vi "基于LabVIEW的多点温度监测系统上位机软件.vi"() -> ()   [LabVIEW 2022 SP3]
uses:
  <vilib>/Instr/_visa.llb/VISA Configure Serial Port (Instr).vi
panel:
  out "获取从机01返回的原始数据包":string
  in  "选择从机":u16(ring)=1 items=["从机01"=1, "从机02"=2]
  out "地址02":dbl[][](graph)
  out "地址01":dbl[][](graph)
  out "提取的第四路温度原始数据":string
  out "提取的第三路温度原始数据":string
  out "提取的第二路温度原始数据":string
  out "提取的第一路温度原始数据":string
  out "提取的第四路温度原始数据":string
  out "提取的第三路温度原始数据":string
  out "提取的第二路温度原始数据":string
  out "提取的第一路温度原始数据":string
  out "第一路温度值":dbl[](array[numeric])
  in  "停止采集":bool
  out "所有测量记录":string[][](table)
  out "第一路温度值":dbl[](array[numeric])
  out "获取从机02返回的原始数据包":string
  in  "发送命令":string
  in  "波特率":u32=9600 caption="波特率(9600)"
  in  "选择串口":refnum<visa-resource-name>
  # "从机地址01："
  # "第二路温度值"
  # "第三路温度值"
  # "第四路温度值"
  # "从机地址02："
  # "第二路温度值"
  # "第三路温度值"
  # "第四路温度值"
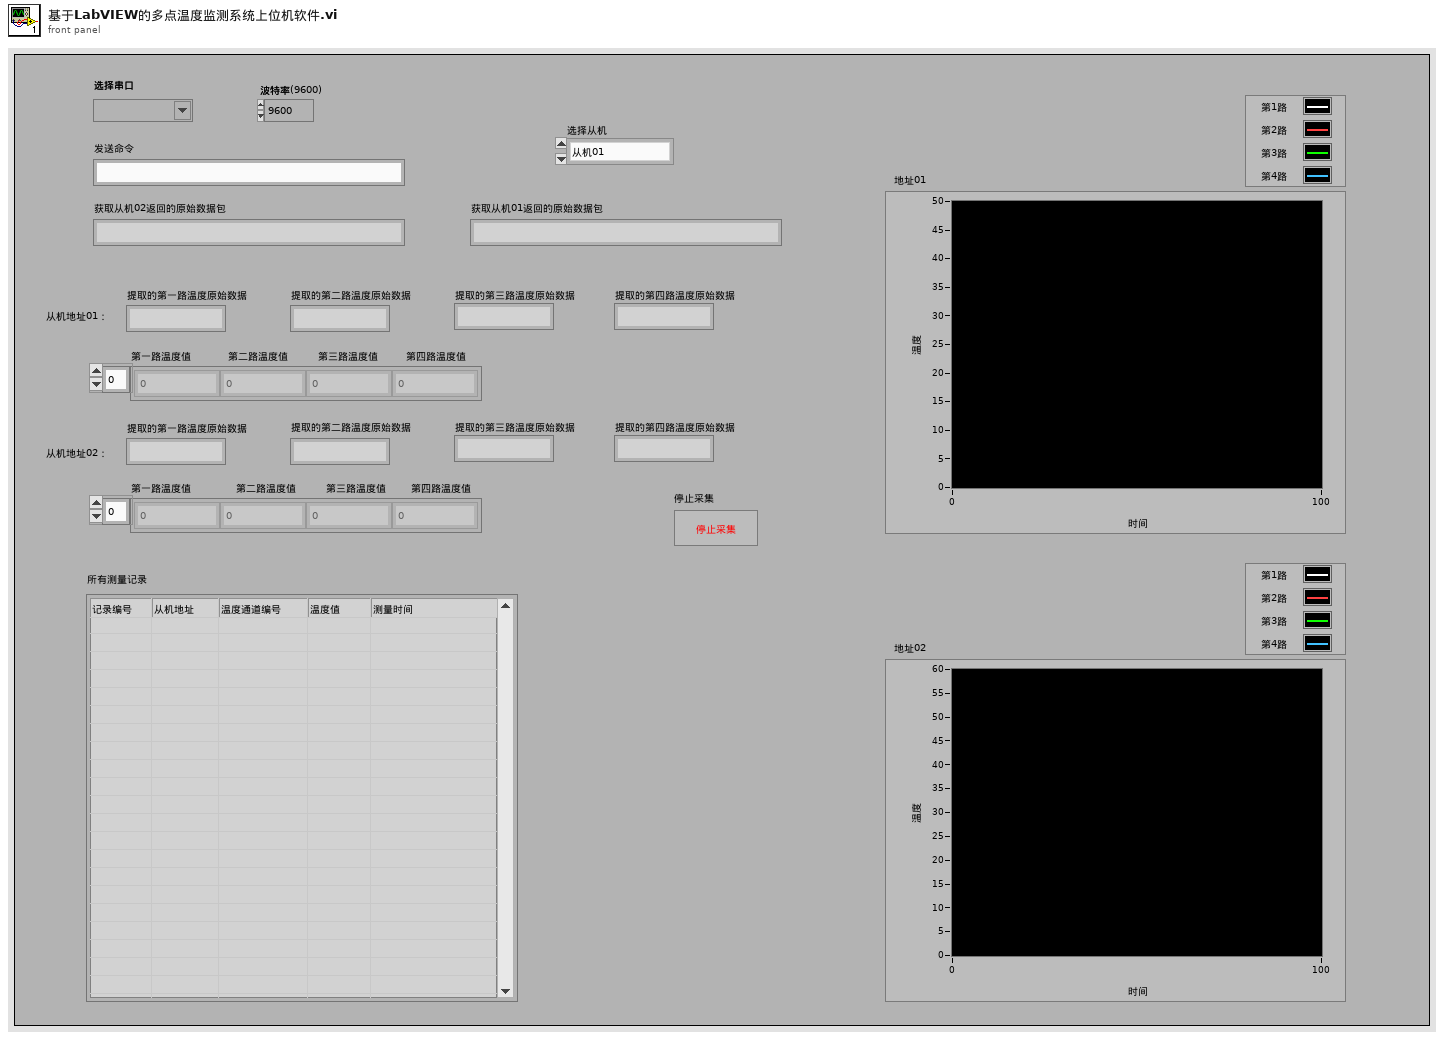
[diagram p1: front panel]
types:
  T1 = typedef "NI_Matrix.lvlib/RealMatrix.ctl" = dbl[][]
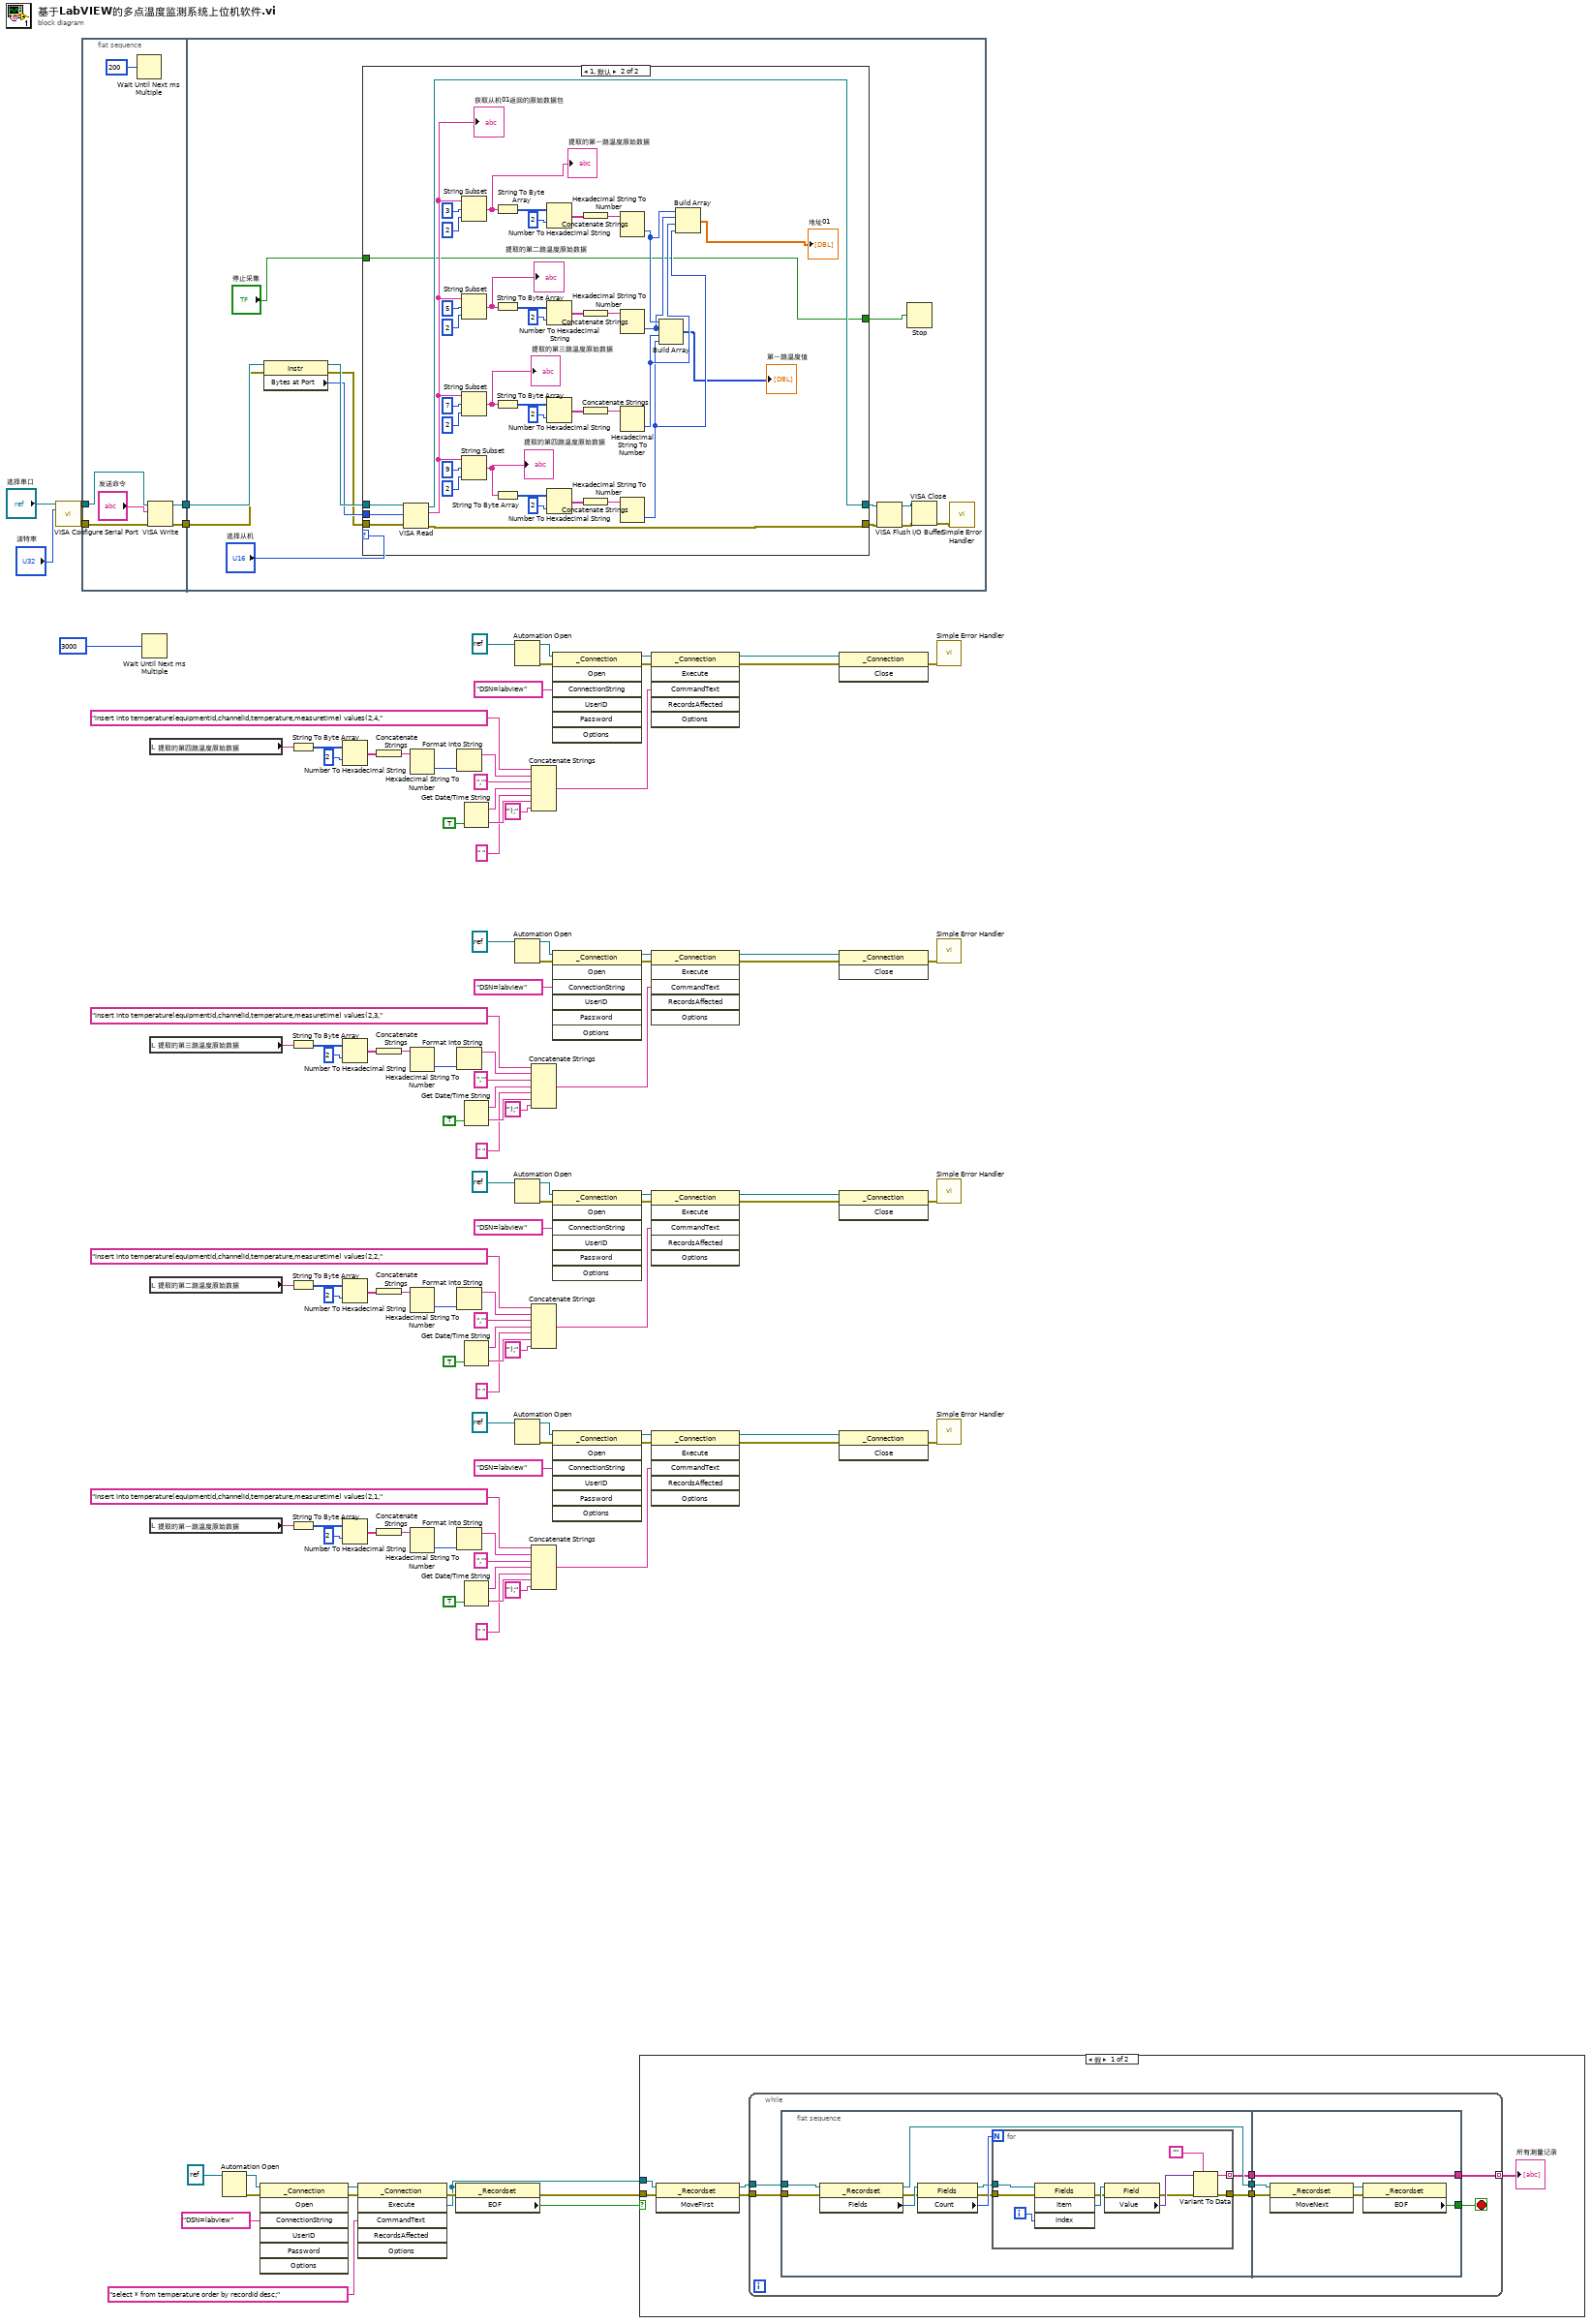
[diagram p0: block diagram]
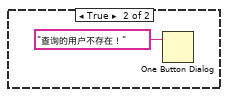
[diagram p2: hidden frame]
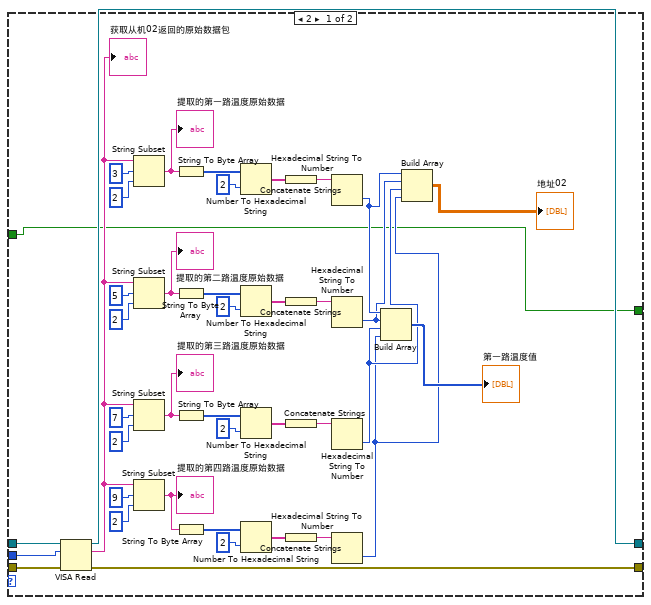
[diagram p3: hidden frame]
diagram:
  n1 = call-poly "VISA Configure Serial Port"("VISA resource name"="选择串口", "baud rate (9600)"="波特率") -> ("VISA resource name out"=w112:refnum<visa-resource-name>, "error out"=w111:errorcluster)  [unwired: 12 in]
  n2 = flat-sequence {
    tunnel: w112 -> [w119]
    tunnel: w111 -> [w118]
    tunnel: [w116] -> w110
    tunnel: [w115] -> w109
    tunnel: w110 -> [w133]
    tunnel: w109 -> [w132]
    frame #0 {
      n3 = Wait Until Next ms Multiple(millisecond multiple=u32 200 ("毫秒倍数")) -> ()  [unwired: 1 out]
      n4 = VISA Write(VISA resource name=w119, write buffer="发送命令", error in (no error)=w118) -> (VISA resource name out=w116:refnum<visa-resource-name>, error out=w115:errorcluster)  [unwired: 1 out]
    }
    frame #1 {
      n5 = property class="Instr"(reference=w133, error in=w132) -> (reference out=w131:refnum<visa-resource-name>, error out=w129:errorcluster, "Bytes at Port"=w130:u32)
      n6 = case shown="1, 默认" "选择从机" {
        tunnel: w131 -> [w174 w178]
        tunnel: w130 -> [w173 w177]
        tunnel: w129 -> [w172 w187]
        tunnel: [w164 w185] -> w125
        tunnel: [w163 w186] -> w124
        tunnel: [w134 w175] -> w121
        tunnel: "停止采集" -> [w134 w175]
        frame 2 {
          n7 = VISA Read(VISA resource name=w174, byte count=w173, error in (no error)=w172) -> (VISA resource name out=w164:refnum<visa-resource-name>, read buffer=w142:string, error out=w163:errorcluster)  [unwired: 1 out]
          "获取从机02返回的原始数据包" <- w142
          n8 = String Subset(string=w142, offset (0)=3 ("偏移量(0)"), length (rest)=2 ("长度（剩余）")) -> (substring=w169:string)
          "提取的第一路温度原始数据" <- w169
          n9 = String Subset(string=w142, offset (0)=5 ("偏移量(0)"), length (rest)=2 ("长度（剩余）")) -> (substring=w160:string)
          "提取的第二路温度原始数据" <- w160
          n10 = String Subset(string=w142, offset (0)=7 ("偏移量(0)"), length (rest)=2 ("长度（剩余）")) -> (substring=w153:string)
          "提取的第三路温度原始数据" <- w153
          n11 = String Subset(string=w142, offset (0)=9 ("偏移量(0)"), length (rest)=2 ("长度（剩余）")) -> (substring=w147:string)
          "提取的第四路温度原始数据" <- w147
          n12 = String To Byte Array(string=w169) -> (unsigned byte array=w168:u8[])
          n13 = String To Byte Array(string=w160) -> (unsigned byte array=w159:u8[])
          n14 = String To Byte Array(string=w153) -> (unsigned byte array=w152:u8[])
          n15 = String To Byte Array(string=w147) -> (unsigned byte array=w146:u8[])
          n16 = Number To Hexadecimal String(1:i16 2 ("宽度(-)"), 2:w168) -> (0:w166:string[])
          n17 = Number To Hexadecimal String(1:i16 2 ("宽度(-)"), 2:w159) -> (0:w157:string[])
          n18 = Number To Hexadecimal String(1:i16 2 ("宽度(-)"), 2:w152) -> (0:w150:string[])
          n19 = Number To Hexadecimal String(1:i16 2 ("宽度(-)"), 2:w146) -> (0:w144:string[])
          n20 = Concatenate Strings(w166) -> (w165:string)
          n21 = Concatenate Strings(w157) -> (w156:string)
          n22 = Concatenate Strings(w150) -> (w149:string)
          n23 = Concatenate Strings(w144) -> (w143:string)
          n24 = Hexadecimal String To Number(string=w165) -> (number=w138:u32)  [unwired: 2 in, 1 out]
          n25 = Hexadecimal String To Number(string=w156) -> (number=w137:u32)  [unwired: 2 in, 1 out]
          n26 = Hexadecimal String To Number(string=w149) -> (number=w136:u32)  [unwired: 2 in, 1 out]
          n27 = Hexadecimal String To Number(string=w143) -> (number=w135:u32)  [unwired: 2 in, 1 out]
          n28 = Build Array(w138, w137, w136, w135) -> (→"第一路温度值":u32[])
          n29 = Build Array(w138, w137, w136, w135) -> (→"地址02":T1)
        }
        frame 1, Default {
          n30 = VISA Read(VISA resource name=w178, byte count=w177, error in (no error)=w187) -> (VISA resource name out=w185:refnum<visa-resource-name>, read buffer=w176:string, error out=w186:errorcluster)  [unwired: 1 out]
          "获取从机01返回的原始数据包" <- w176
          n31 = String Subset(string=w176, offset (0)=3 ("偏移量(0)"), length (rest)=2 ("长度（剩余）")) -> (substring=w181:string)
          "提取的第一路温度原始数据" <- w181
          n32 = String Subset(string=w176, offset (0)=5 ("偏移量(0)"), length (rest)=2 ("长度（剩余）")) -> (substring=w182:string)
          "提取的第二路温度原始数据" <- w182
          n33 = String Subset(string=w176, offset (0)=7 ("偏移量(0)"), length (rest)=2 ("长度（剩余）")) -> (substring=w183:string)
          "提取的第三路温度原始数据" <- w183
          n34 = String Subset(string=w176, offset (0)=9 ("偏移量(0)"), length (rest)=2 ("长度（剩余）")) -> (substring=w184:string)
          "提取的第四路温度原始数据" <- w184
          n35 = String To Byte Array(string=w181) -> (unsigned byte array=w213:u8[])
          n36 = String To Byte Array(string=w182) -> (unsigned byte array=w207:u8[])
          n37 = String To Byte Array(string=w183) -> (unsigned byte array=w201:u8[])
          n38 = String To Byte Array(string=w184) -> (unsigned byte array=w196:u8[])
          n39 = Number To Hexadecimal String(1:i16 2 ("宽度(-)"), 2:w213) -> (0:w211:string[])
          n40 = Number To Hexadecimal String(1:i16 2 ("宽度(-)"), 2:w207) -> (0:w205:string[])
          n41 = Number To Hexadecimal String(1:i16 2 ("宽度(-)"), 2:w201) -> (0:w199:string[])
          n42 = Number To Hexadecimal String(1:i16 2 ("宽度(-)"), 2:w196) -> (0:w194:string[])
          n43 = Concatenate Strings(w211) -> (w210:string)
          n44 = Concatenate Strings(w205) -> (w204:string)
          n45 = Concatenate Strings(w199) -> (w198:string)
          n46 = Concatenate Strings(w194) -> (w193:string)
          n47 = Hexadecimal String To Number(string=w210) -> (number=w191:u32)  [unwired: 2 in, 1 out]
          n48 = Hexadecimal String To Number(string=w204) -> (number=w190:u32)  [unwired: 2 in, 1 out]
          n49 = Hexadecimal String To Number(string=w198) -> (number=w189:u32)  [unwired: 2 in, 1 out]
          n50 = Hexadecimal String To Number(string=w193) -> (number=w188:u32)  [unwired: 2 in, 1 out]
          n51 = Build Array(w191, w190, w189, w188) -> (→"第一路温度值":u32[])
          n52 = Build Array(w191, w190, w189, w188) -> (→"地址01":T1)
        }
      }
      n53 = VISA Flush I/O Buffer(VISA resource name=w125, error in (no error)=w124) -> (VISA resource name out=w126:refnum<visa-resource-name>, error out=w127:errorcluster)  [unwired: 1 in]
      n54 = Stop(stop? (T)=w121) -> ()
      n55 = VISA Close(VISA resource name=w126, error in (no error)=w127) -> (error out=w128:errorcluster)
      n56 = call <vilib>:"Simple Error Handler.vi"("error in (no error)"=w128) -> ()  [unwired: 4 in, 5 out]
    }
  }
  n57 = Wait Until Next ms Multiple(millisecond multiple=3000) -> ()  [unwired: 1 out]
  n58 = local read "提取的第四路温度原始数据"() -> (w2:string)
  n59 = local read "提取的第三路温度原始数据"() -> (w3:string)
  n60 = local read "提取的第二路温度原始数据"() -> (w44:string)
  n61 = local read "提取的第一路温度原始数据"() -> (w65:string)
  n62 = Automation Open(Automation Refnum=refnum<k7> refnum ("ADODB._Connection")) -> (Automation Refnum=w107:refnum<k7>, error out=w106:errorcluster)  [unwired: 3 in]
  n63 = invoke class="_Connection" method="Open"(reference=w107, error in=w106, "ConnectionString"="DSN=labview") -> (reference out=w104:refnum<k7>, error out=w103:errorcluster)  [unwired: 4 in, 5 out]
  n64 = String To Byte Array(string=w2) -> (unsigned byte array=w20:u8[])
  n65 = String To Byte Array(string=w3) -> (unsigned byte array=w40:u8[])
  n66 = String To Byte Array(string=w44) -> (unsigned byte array=w61:u8[])
  n67 = String To Byte Array(string=w65) -> (unsigned byte array=w82:u8[])
  n68 = Number To Hexadecimal String(1:i16 2 ("宽度(-)"), 2:w20) -> (0:w21:string[])
  n69 = Number To Hexadecimal String(1:i16 2 ("宽度(-)"), 2:w40) -> (0:w41:string[])
  n70 = Number To Hexadecimal String(1:i16 2 ("宽度(-)"), 2:w61) -> (0:w62:string[])
  n71 = Number To Hexadecimal String(1:i16 2 ("宽度(-)"), 2:w82) -> (0:w83:string[])
  n72 = invoke class="_Connection" method="Execute"(reference=w104, error in=w103, "CommandText"="select * from temperature order by recordid desc;") -> (error out=w101:errorcluster, "Execute"=w99:refnum<k7>)  [unwired: 3 in, 4 out]
  n73 = Concatenate Strings(w21) -> (w22:string)
  n74 = Concatenate Strings(w41) -> (w42:string)
  n75 = Concatenate Strings(w62) -> (w63:string)
  n76 = Concatenate Strings(w83) -> (w84:string)
  n77 = Hexadecimal String To Number(string=w22) -> (number=w23:u32)  [unwired: 2 in, 1 out]
  n78 = Hexadecimal String To Number(string=w42) -> (number=w43:u32)  [unwired: 2 in, 1 out]
  n79 = Hexadecimal String To Number(string=w63) -> (number=w64:u32)  [unwired: 2 in, 1 out]
  n80 = Hexadecimal String To Number(string=w84) -> (number=w85:u32)  [unwired: 2 in, 1 out]
  n81 = property class="_Recordset"(reference=w99, error in=w101) -> (error out=w98:errorcluster, "EOF"=w100:bool)  [unwired: 1 out]
  n82 = Format Into String(w23) -> (resulting string=w19:string)  [unwired: 3 in, 1 out]
  n83 = Format Into String(w43) -> (resulting string=w39:string)  [unwired: 3 in, 1 out]
  n84 = Format Into String(w64) -> (resulting string=w60:string)  [unwired: 3 in, 1 out]
  n85 = Format Into String(w85) -> (resulting string=w81:string)  [unwired: 3 in, 1 out]
  n86 = Get Date/Time String(want seconds? (F)=TRUE) -> (date string=w12:string, time string=w13:string)  [unwired: 2 in]
  n87 = Get Date/Time String(want seconds? (F)=TRUE) -> (date string=w32:string, time string=w33:string)  [unwired: 2 in]
  n88 = Get Date/Time String(want seconds? (F)=TRUE) -> (date string=w53:string, time string=w54:string)  [unwired: 2 in]
  n89 = Get Date/Time String(want seconds? (F)=TRUE) -> (date string=w74:string, time string=w75:string)  [unwired: 2 in]
  n90 = Automation Open(Automation Refnum=refnum<k7> refnum ("ADODB._Connection")) -> (Automation Refnum=w18:refnum<k7>, error out=w17:errorcluster)  [unwired: 3 in]
  n91 = Automation Open(Automation Refnum=refnum<k7> refnum ("ADODB._Connection")) -> (Automation Refnum=w38:refnum<k7>, error out=w37:errorcluster)  [unwired: 3 in]
  n92 = Automation Open(Automation Refnum=refnum<k7> refnum ("ADODB._Connection")) -> (Automation Refnum=w59:refnum<k7>, error out=w58:errorcluster)  [unwired: 3 in]
  n93 = Automation Open(Automation Refnum=refnum<k7> refnum ("ADODB._Connection")) -> (Automation Refnum=w80:refnum<k7>, error out=w79:errorcluster)  [unwired: 3 in]
  n94 = Concatenate Strings("insert into temperature(equipmentid,channelid,temperature,measuretime) values(2,4," ("CommandText"), w19, ",'" ("字符串"), w12, " " ("string"), w13, "');" ("string")) -> (w14:string)
  n95 = Concatenate Strings("insert into temperature(equipmentid,channelid,temperature,measuretime) values(2,3," ("CommandText"), w39, ",'" ("字符串"), w32, " " ("string"), w33, "');" ("string")) -> (w34:string)
  n96 = Concatenate Strings("insert into temperature(equipmentid,channelid,temperature,measuretime) values(2,2," ("CommandText"), w60, ",'" ("字符串"), w53, " " ("string"), w54, "');" ("string")) -> (w55:string)
  n97 = Concatenate Strings("insert into temperature(equipmentid,channelid,temperature,measuretime) values(2,1," ("CommandText"), w81, ",'" ("字符串"), w74, " " ("string"), w75, "');" ("string")) -> (w76:string)
  n98 = invoke class="_Connection" method="Open"(reference=w18, error in=w17, "ConnectionString"="DSN=labview") -> (reference out=w16:refnum<k7>, error out=w15:errorcluster)  [unwired: 4 in, 5 out]
  n99 = invoke class="_Connection" method="Open"(reference=w38, error in=w37, "ConnectionString"="DSN=labview") -> (reference out=w36:refnum<k7>, error out=w35:errorcluster)  [unwired: 4 in, 5 out]
  n100 = invoke class="_Connection" method="Open"(reference=w59, error in=w58, "ConnectionString"="DSN=labview") -> (reference out=w57:refnum<k7>, error out=w56:errorcluster)  [unwired: 4 in, 5 out]
  n101 = invoke class="_Connection" method="Open"(reference=w80, error in=w79, "ConnectionString"="DSN=labview") -> (reference out=w78:refnum<k7>, error out=w77:errorcluster)  [unwired: 4 in, 5 out]
  n102 = case shown="假" w100 {
    tunnel: w99 -> [w220 _]
    tunnel: w98 -> [w219 _]
    frame False {
      n103 = invoke class="_Recordset" method="MoveFirst"(reference=w220, error in=w219) -> (reference out=w217:refnum<k7>, error out=w218:errorcluster)  [unwired: 1 in, 1 out]
      n104 = while {
        tunnel: w218 -> [w225]
        tunnel: w217 -> [w224]
        tunnel: [w221] -> w216 mode=indexing
        stop <- w223 stop-if-true
        n105 = flat-sequence {
          tunnel: w224 -> [w237]
          tunnel: w225 -> [w236]
          tunnel: [w230] -> w227
          tunnel: [w229] -> w226
          tunnel: [w228] -> w222
          tunnel: w227 -> [w251]
          tunnel: w226 -> [w250]
          tunnel: [w249] -> w223
          tunnel: w222 -> [w248]
          tunnel: [w248] -> w221
          frame #0 {
            n106 = property class="_Recordset"(reference=w237, error in=w236) -> (reference out=w229:refnum<k7>, error out=w234:errorcluster, "Fields"=w235:refnum<k7>)
            n107 = property class="Fields"(reference=w235, error in=w234) -> (reference out=w232:refnum<k7>, error out=w231:errorcluster, "Count"=w233:i32)
            n108 = for {
              N: w233 -> [_]
              tunnel: w232 -> [w242]
              tunnel: w231 -> [w241]
              tunnel: [w239] -> w228 mode=indexing
              tunnel: [w238] -> w230
              i -> [w240]
              n109 = invoke class="Fields" method="Item"(reference=w242, error in=w241, "Index"=w240) -> (error out=w246:errorcluster, "Item"=w247:refnum<k7>)  [unwired: 1 in, 2 out]
              n110 = property class="Field"(reference=w247, error in=w246) -> (error out=w243:errorcluster, "Value"=w244:variant)  [unwired: 1 out]
              n111 = Variant To Data(error in=w243, type="", Variant=w244) -> (data=w239:string, error out=w238:errorcluster)
            }
          }
          frame #1 {
            n112 = invoke class="_Recordset" method="MoveNext"(reference=w250, error in=w251) -> (reference out=w253:refnum<k7>, error out=w252:errorcluster)  [unwired: 1 in, 1 out]
            n113 = property class="_Recordset"(reference=w253, error in=w252) -> ("EOF"=w249:bool)  [unwired: 2 out]
          }
        }
      }
      "所有测量记录" <- w216
    }
    frame True {
      n114 = One Button Dialog(message="查询的用户不存在！") -> ()  [unwired: 1 in, 1 out]
    }
  }
  n115 = invoke class="_Connection" method="Execute"(reference=w16, error in=w15, "CommandText"=w14) -> (reference out=w87:refnum<k7>, error out=w86:errorcluster)  [unwired: 3 in, 4 out]
  n116 = invoke class="_Connection" method="Execute"(reference=w36, error in=w35, "CommandText"=w34) -> (reference out=w90:refnum<k7>, error out=w89:errorcluster)  [unwired: 3 in, 4 out]
  n117 = invoke class="_Connection" method="Execute"(reference=w57, error in=w56, "CommandText"=w55) -> (reference out=w93:refnum<k7>, error out=w92:errorcluster)  [unwired: 3 in, 4 out]
  n118 = invoke class="_Connection" method="Execute"(reference=w78, error in=w77, "CommandText"=w76) -> (reference out=w96:refnum<k7>, error out=w95:errorcluster)  [unwired: 3 in, 4 out]
  n119 = invoke class="_Connection" method="Close"(reference=w87, error in=w86) -> (error out=w88:errorcluster)  [unwired: 1 in, 2 out]
  n120 = invoke class="_Connection" method="Close"(reference=w90, error in=w89) -> (error out=w91:errorcluster)  [unwired: 1 in, 2 out]
  n121 = invoke class="_Connection" method="Close"(reference=w93, error in=w92) -> (error out=w94:errorcluster)  [unwired: 1 in, 2 out]
  n122 = invoke class="_Connection" method="Close"(reference=w96, error in=w95) -> (error out=w97:errorcluster)  [unwired: 1 in, 2 out]
  n123 = call <vilib>:"Simple Error Handler.vi"("error in (no error)"=w88) -> ()  [unwired: 4 in, 5 out]
  n124 = call <vilib>:"Simple Error Handler.vi"("error in (no error)"=w91) -> ()  [unwired: 4 in, 5 out]
  n125 = call <vilib>:"Simple Error Handler.vi"("error in (no error)"=w94) -> ()  [unwired: 4 in, 5 out]
  n126 = call <vilib>:"Simple Error Handler.vi"("error in (no error)"=w97) -> ()  [unwired: 4 in, 5 out]
